vi "SPI_launcher.vi"   [LabVIEW 2023]
uses:
  <vilib>/ActorFramework/Actor/Actor.lvclass
  SinglePhotonInterferenceUI.lvclass
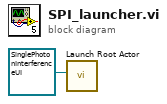
[diagram p0: block diagram]
diagram:
  n1 = call <vilib>:"Launch Root Actor.vi"("Actor"=refnum<class "SinglePhotonInterferenceUI.lvclass"> refnum ("SinglePhotonInterferenceUI.lvlib:SinglePhotonInterferenceUI.lvclass")) -> ()  [unwired: 9 in, 2 out]
